vi "Hybrid PS Control Gateway.vi"() -> ()   [LabVIEW 2020]
panel:
  in  "Slew Rate":dbl caption="[A/s]\n(0.0) Max)" step=1e-05 format="%.5f"
  in  "stop":bool
  in  "Pause":bool
  in  "Ramp":bool
  in  "Setpoint":dbl caption="[kA]\n(0.0) Max)" step=1e-05 format="%.5f"
  # "(To Zero Goes\nTo 100 A)"
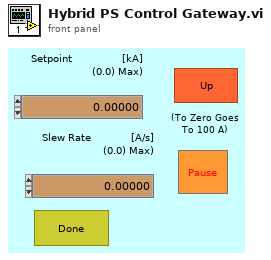
[diagram p1: front panel]
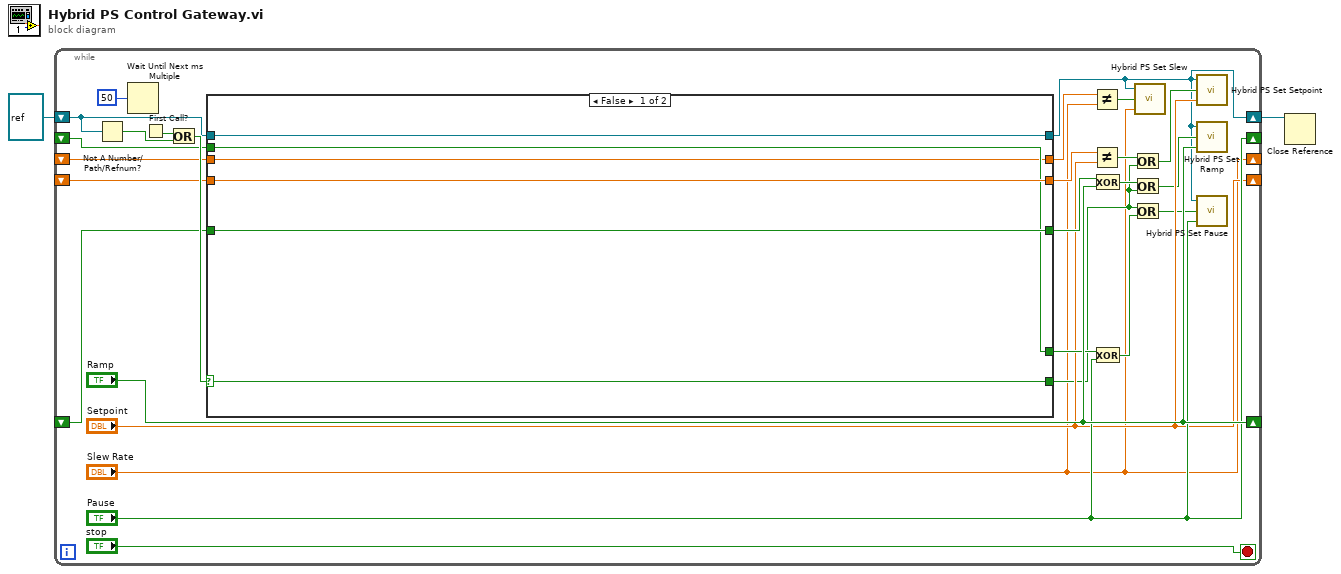
[diagram p0: block diagram]
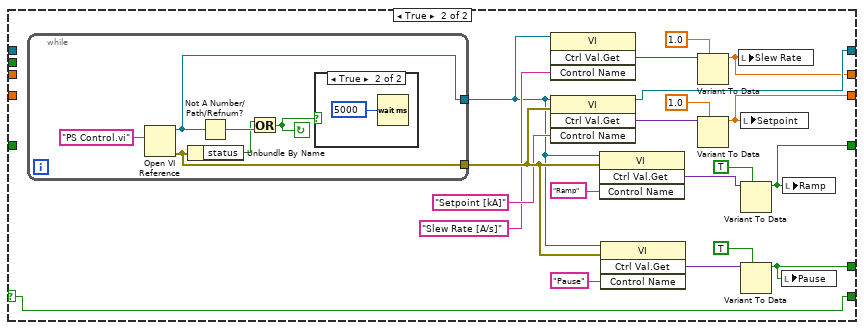
[diagram p2: hidden frame]
diagram:
  n1 = while {
    shift-left: _ -> [w15]
    shift-right: ["Pause"] -> _
    shift-left: _ -> [w17]
    shift-right: ["Ramp"] -> _
    shift-left: _ -> [w19]
    shift-right: ["Setpoint"] -> _
    shift-right: [w5] -> w1
    shift-left: refnum<vi> refnum -> [w20]
    shift-right: ["Slew Rate"] -> _
    shift-left: _ -> [w4]
    stop <- "stop" stop-if-true
    n2 = Not A Number/Path/Refnum?(number/path/refnum=w20) -> (NaN/Path/Refnum?=w23:bool)
    n3 = Wait Until Next ms Multiple(millisecond multiple=u32 50) -> ()  [unwired: 1 out]
    n4 = First Call?() -> (First Call?: T/F=w22:bool)
    n5 = Or(x=w22, y=w23) -> (x .or. y?=w21:bool)
    n6 = case shown="False" w21 {
      selector: w21 -> [w31 w41]
      tunnel: w20 -> [w35 _]
      tunnel: [w35 w51] -> w5
      tunnel: [w34 w49] -> w18
      tunnel: w19 -> [w34 _]
      tunnel: [w33 w47] -> w16
      tunnel: w17 -> [w33 _]
      tunnel: [w32 w43] -> w14
      tunnel: w15 -> [w32 _]
      tunnel: [w31 w41] -> w8
      tunnel: [w30 w36] -> w7
      tunnel: w4 -> [w30 _]
      frame False {
      }
      frame True {
        n7 = while {
          tunnel: [w59] -> w37
          tunnel: [w58] -> w54
          stop <- w56 continue-if-true
          n8 = Open VI Reference(vi path="PS Control.vi") -> (vi reference=w59:refnum<vi>, error out=w58:errorcluster)  [unwired: 5 in]
          n9 = Unbundle By Name(w58) -> ("status"=w57:bool)
          n10 = Not A Number/Path/Refnum?(number/path/refnum=w59) -> (NaN/Path/Refnum?=w60:bool)
          n11 = Or(x=w57, y=w60) -> (x .or. y?=w56:bool)
          n12 = case shown="True" w56 {
            frame False {
            }
            frame True {
              n13 = Wait (ms)(milliseconds to wait=u32 5000) -> ()  [unwired: 1 out]
            }
          }
        }
        n14 = invoke class="VI" method="Ctrl Val.Get"(reference=w37, "Control Name"="Slew Rate [A/s]") -> ("Get Control Value Variant"=w39:variant)  [unwired: 2 in, 3 out]
        n15 = invoke class="VI" method="Ctrl Val.Get"(reference=w37, error in=w54, "Control Name"="Setpoint [kA]") -> (reference out=w51:refnum<vi>, "Get Control Value Variant"=w50:variant)  [unwired: 1 in, 2 out]
        n16 = invoke class="VI" method="Ctrl Val.Get"(reference=w37, error in=w54, "Control Name"="Ramp") -> ("Get Control Value Variant"=w48:variant)  [unwired: 1 in, 3 out]
        n17 = invoke class="VI" method="Ctrl Val.Get"(reference=w37, error in=w54, "Control Name"="Pause") -> ("Get Control Value Variant"=w44:variant)  [unwired: 1 in, 3 out]
        n18 = Variant To Data(type=1.0, Variant=w39) -> (data=w36:dbl)  [unwired: 1 in, 1 out]
        n19 = Variant To Data(type=1.0, Variant=w50) -> (data=w49:dbl)  [unwired: 1 in, 1 out]
        n20 = local write "Slew Rate"(w36) -> ()
        n21 = local write "Setpoint"(w49) -> ()
        n22 = Variant To Data(type=TRUE, Variant=w48) -> (data=w47:bool)  [unwired: 1 in, 1 out]
        n23 = Variant To Data(type=TRUE, Variant=w44) -> (data=w43:bool)  [unwired: 1 in, 1 out]
        n24 = local write "Pause"(w43) -> ()
        n25 = local write "Ramp"(w47) -> ()
      }
    }
    n26 = Not Equal?(x=w7, y="Slew Rate") -> (x != y?=w6:bool)
    n27 = Not Equal?(x=w18, y="Setpoint") -> (x != y?=w13:bool)
    n28 = Exclusive Or(1:"Ramp", 2:w16) -> (0:w27:bool)
    n29 = Exclusive Or(1:"Pause", 2:w14) -> (0:w26:bool)
    n30 = Or(x=w13, y=w8) -> (x .or. y?=w9:bool)
    n31 = Or(x=w27, y=w8) -> (x .or. y?=w10:bool)
    n32 = Or(x=w8, y=w26) -> (x .or. y?=w11:bool)
    n33 = call "Hybrid PS Set Slew.vi"("Slew Rate"="Slew Rate", "Change it"=w6, "VI Refnum"=w5) -> ()
    n34 = call "Hybrid PS Set Setpoint.vi"("Setpoint"="Setpoint", "Change it"=w9, "VI Refnum"=w5) -> ()
    n35 = call "Hybrid PS Set Ramp.vi"("Ramp"="Ramp", "Change it"=w10, "VI Refnum"=w5) -> ()
    n36 = call "Hybrid PS Set Pause.vi"("Pause"="Pause", "Change it"=w11, "VI Refnum"=w5) -> ()
  }
  n37 = Close Reference(reference=w1) -> ()  [unwired: 1 in, 1 out]
